vi "Store_Val_CH2.vi"(8 "Store":bool, 11 "Vin":dbl) -> (3 "Saved Value":dbl)   [LabVIEW 2012]
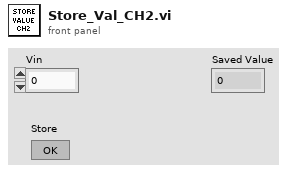
[diagram p1: front panel]
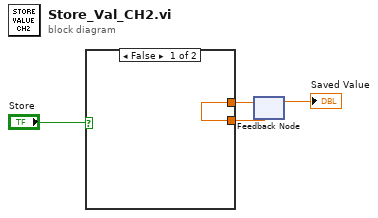
[diagram p0: block diagram]
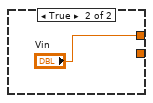
[diagram p2: hidden frame]
diagram:
  n1 = feedback #1() -> (w1:dbl)  [unwired: 1 in]
  "Saved Value" <- w1
  n2 = case shown="False" "Store" {
    tunnel: [w4 "Vin"] -> w2
    tunnel: w1 -> [w4 _]
    frame False {
    }
    frame True {
    }
  }
  n3 = feedback-in #1(w2) -> ()
